vi "main.vi"() -> ()   [LabVIEW 2010]
uses:
  scan_specification_tagResonant.ctl
  common_typedefs/DAC_voltage_tagResonantr.ctl
  FPGA tracking/polar tracking settings.ctl
  FPGA tracking/spot location constraints.ctl
  FPGA tracking/spot location constraint.ctl
  FPGA tracking/kalman N spot state.ctl
  counter_cluster_tagResonant.ctl
  integration_cluster.ctl
  common_typedefs/channels_cluster.ctl
  FPGA tracking/kalman pv state.ctl
  FPGA tracking/control flags.ctl
  <vilib>/Platform/TimedLoop/XDataNode/XDataNode.xnode
  <vilib>/Platform/TimedLoop/XDataNode/timing_clust.ctl
  <vilib>/Platform/TimedLoop/XDataNode/nitl_modes.ctl
  <vilib>/Platform/TimedLoop/XDataNode/wakeup.ctl
  <vilib>/rvi/FXPMathLib/FxpMul/XNode/nifxpmath_Multiplier.xnode
  <vilib>/rvi/FXPMathLib/FxpMul/subVIs/nifxpmath_Mul_SimConfig.ctl
  <vilib>/fxp/LVFixedPointQuantizationPolicyTypeDef.ctl
  <vilib>/fxp/LVFixedPointOverflowPolicyTypeDef.ctl
  <vilib>/eio/EIONode/EIONode.xnode
  <vilib>/rvi/eio/nirviEIOImplementation/nirviEIOImplementation.xnode
  <vilib>/rvi/eio/common/nirviEmuClasses.ctl
  <vilib>/rvi/DataTransferAndStorage/Container/XNode/niFpgaContainer.xnode
  FPGA scanInfo/scan message.ctl
  <vilib>/rvi/DataTransferAndStorage/Container/Common/niFpgaContainerMethod.ctl
  <vilib>/rvi/DataTransferAndStorage/Container/Common/niFpgaTransferTypeControl.ctl
  <vilib>/rvi/FXPMathLib/FxpMul/simVIs/DllFxpMulTemp_sub.vi
  <vilib>/rvi/eio/common/nirviEmuTemplateMethod_noerrors.vi
  <vilib>/rvi/FIFO/Fifo_Resource/nirvififoEmulationSetSize.vi
  <vilib>/rvi/DataTransferAndStorage/Container/Common/niFpgaContainerGetUniqueNameForEmu.vi
  <vilib>/rvi/interface/RandomDataEmulation/nirviRandomDataFPGAFIFO.vi
  <vilib>/rvi/interface/RandomDataEmulation/niFpgaRandomDataHandleErrors.vi
  <vilib>/Platform/TimedLoop/XDataNode/XDNodeRunTimeDep.lvlib
panel:
  in  "total cycles per stim cycle":u16
  in  "lines per stim":u16
  in  "stim by cycle":bool
  in  "stim delay":i16=5
  in  "bleach mode":bool
  in  "pockels always on":bool
  in  "invert optog stim":bool
  in  "optog all spots":bool
  in  "optog target spot":u8
  in  "ff vel?":bool
  out "N spot tracker out":T1
  in  "spot location constraints":T2=[{"spot number"=0, "active"=FALSE, "x max"=0, "x min"=0, "y max"=0, "y min"=0}, {"spot number"=0, "active"=FALSE, "x max"=0, "x min"=0, "y max"=0, "y min"=0}, {"spot number"=0, "active"=FALSE, "x max"=0, "x min"=0, "y max"=0, "y min"=0}, {"spot number"=0, "active"=FALSE, "x max"=0, "x min"=0, "y max"=0, "y min"=0}]
  in  "reset flags":u8
  in  "mark valid location":bool
  out "Spot locations":T4(array[cluster])
  in  "inter-spot delay":u8
  in  "circles per spot":u16
  in  "number of spots":u8
  in  "stim buffer counts":u16=20
  in  "TAG slice options":T5
  out "n photons during stim":u32
  out "stim time":u32
  in  "stimulus on (low f)":bool=TRUE
  out "y-offset":i16
  out "x-offset":i16
  in  "measure offset":bool
  in  "Vxy feedback":bool
  out "piezo z-offset":i16
  in  "piezoToTrackingScale":fxp<+/-,16,2>
  out "piezo out":i16
  in  "piezo z feedback":bool
  in  "trackingToPiezoScale":fxp<+/-,16,5> format="%.16g"
  out "z-location":i16
  in  "Vz feedback?":bool
  in  "half valid z-range (ncycles * 64)":i16=500
  in  "x-y phase shift (*2^16/2*pi)":u16=16384
  in  "vmax":fxp<+,16,0>=0.0016021728515625 format="%.32g"
  in  "tracking settings":T6
  out "AI values":u32
  in  "min photons for update":u32=200
  out "pixels sent":u32
  out "lines sent":u32
  in  "tracking?":bool
  in  "feedback channel":enum16{"channel 0", "channel 1", "both"}(ring)=enum."both"
  out "ticks for AI read":u32
  in  "AI look-ahead":i16
  out "ticks to transmit":i32
  in  "useReadPosition":bool
  out "DAC voltages":T7 {"pockels" max=4095 step=1; "y" max=4095 step=1; "x" max=4095 step=1}
  in  "scan specification":T8={"z resolution (pixels)"=1000, "iterations per pixel"=28, "iterations per z-scan (=zres*iterperpixel)"=50, "x resolution (pixels)"=100, "y resolution (pixels)"=80, "number of z-lines per volume"=30, "number of repetitions (volumes)"=5, "Pockels cell voltage (bits)"=-1, "Vx center (bits)"=0, "Vy center (bits)"=0, "Vx amplitude (bits)"=40, "Vy amplitude (bits)"=0, "lines to delay between scan start and output"=1, "LSB has acquire control"=FALSE, "Pockels cell bleach voltage"=0}
  out "FIFO overflow":bool
  in  "scan":bool
  in  "stop":bool
  in  "stop acquisition at\nFIFO overflow?":bool
  out "scanning?":bool
  # "Mirna: \niterations per pixel = (x scan segment fraction*fFPGA)/(x resolution*f resonance)\nfFPGA/f resonance = 5000 --assumes 8kHz resonance frequency\niterations per pixel=25"
  # "used to be 1000 (Mirna)"
  # "to control how line locations are found"
  # "y settings:\ny resolution*y step size = 6553\nthis gives scan from -1 to 1V\ny resolution = 200\ny step size = 33\n\nz settings:\nto scan entire y profile \nnumber of z's has to be equal\ny resolution"
  # "1. use ftn generators to test galvo inputs\n2. right now AI+ and AI- == differential configuration\nThere is also an option AI+ and GND = referenced single ended"
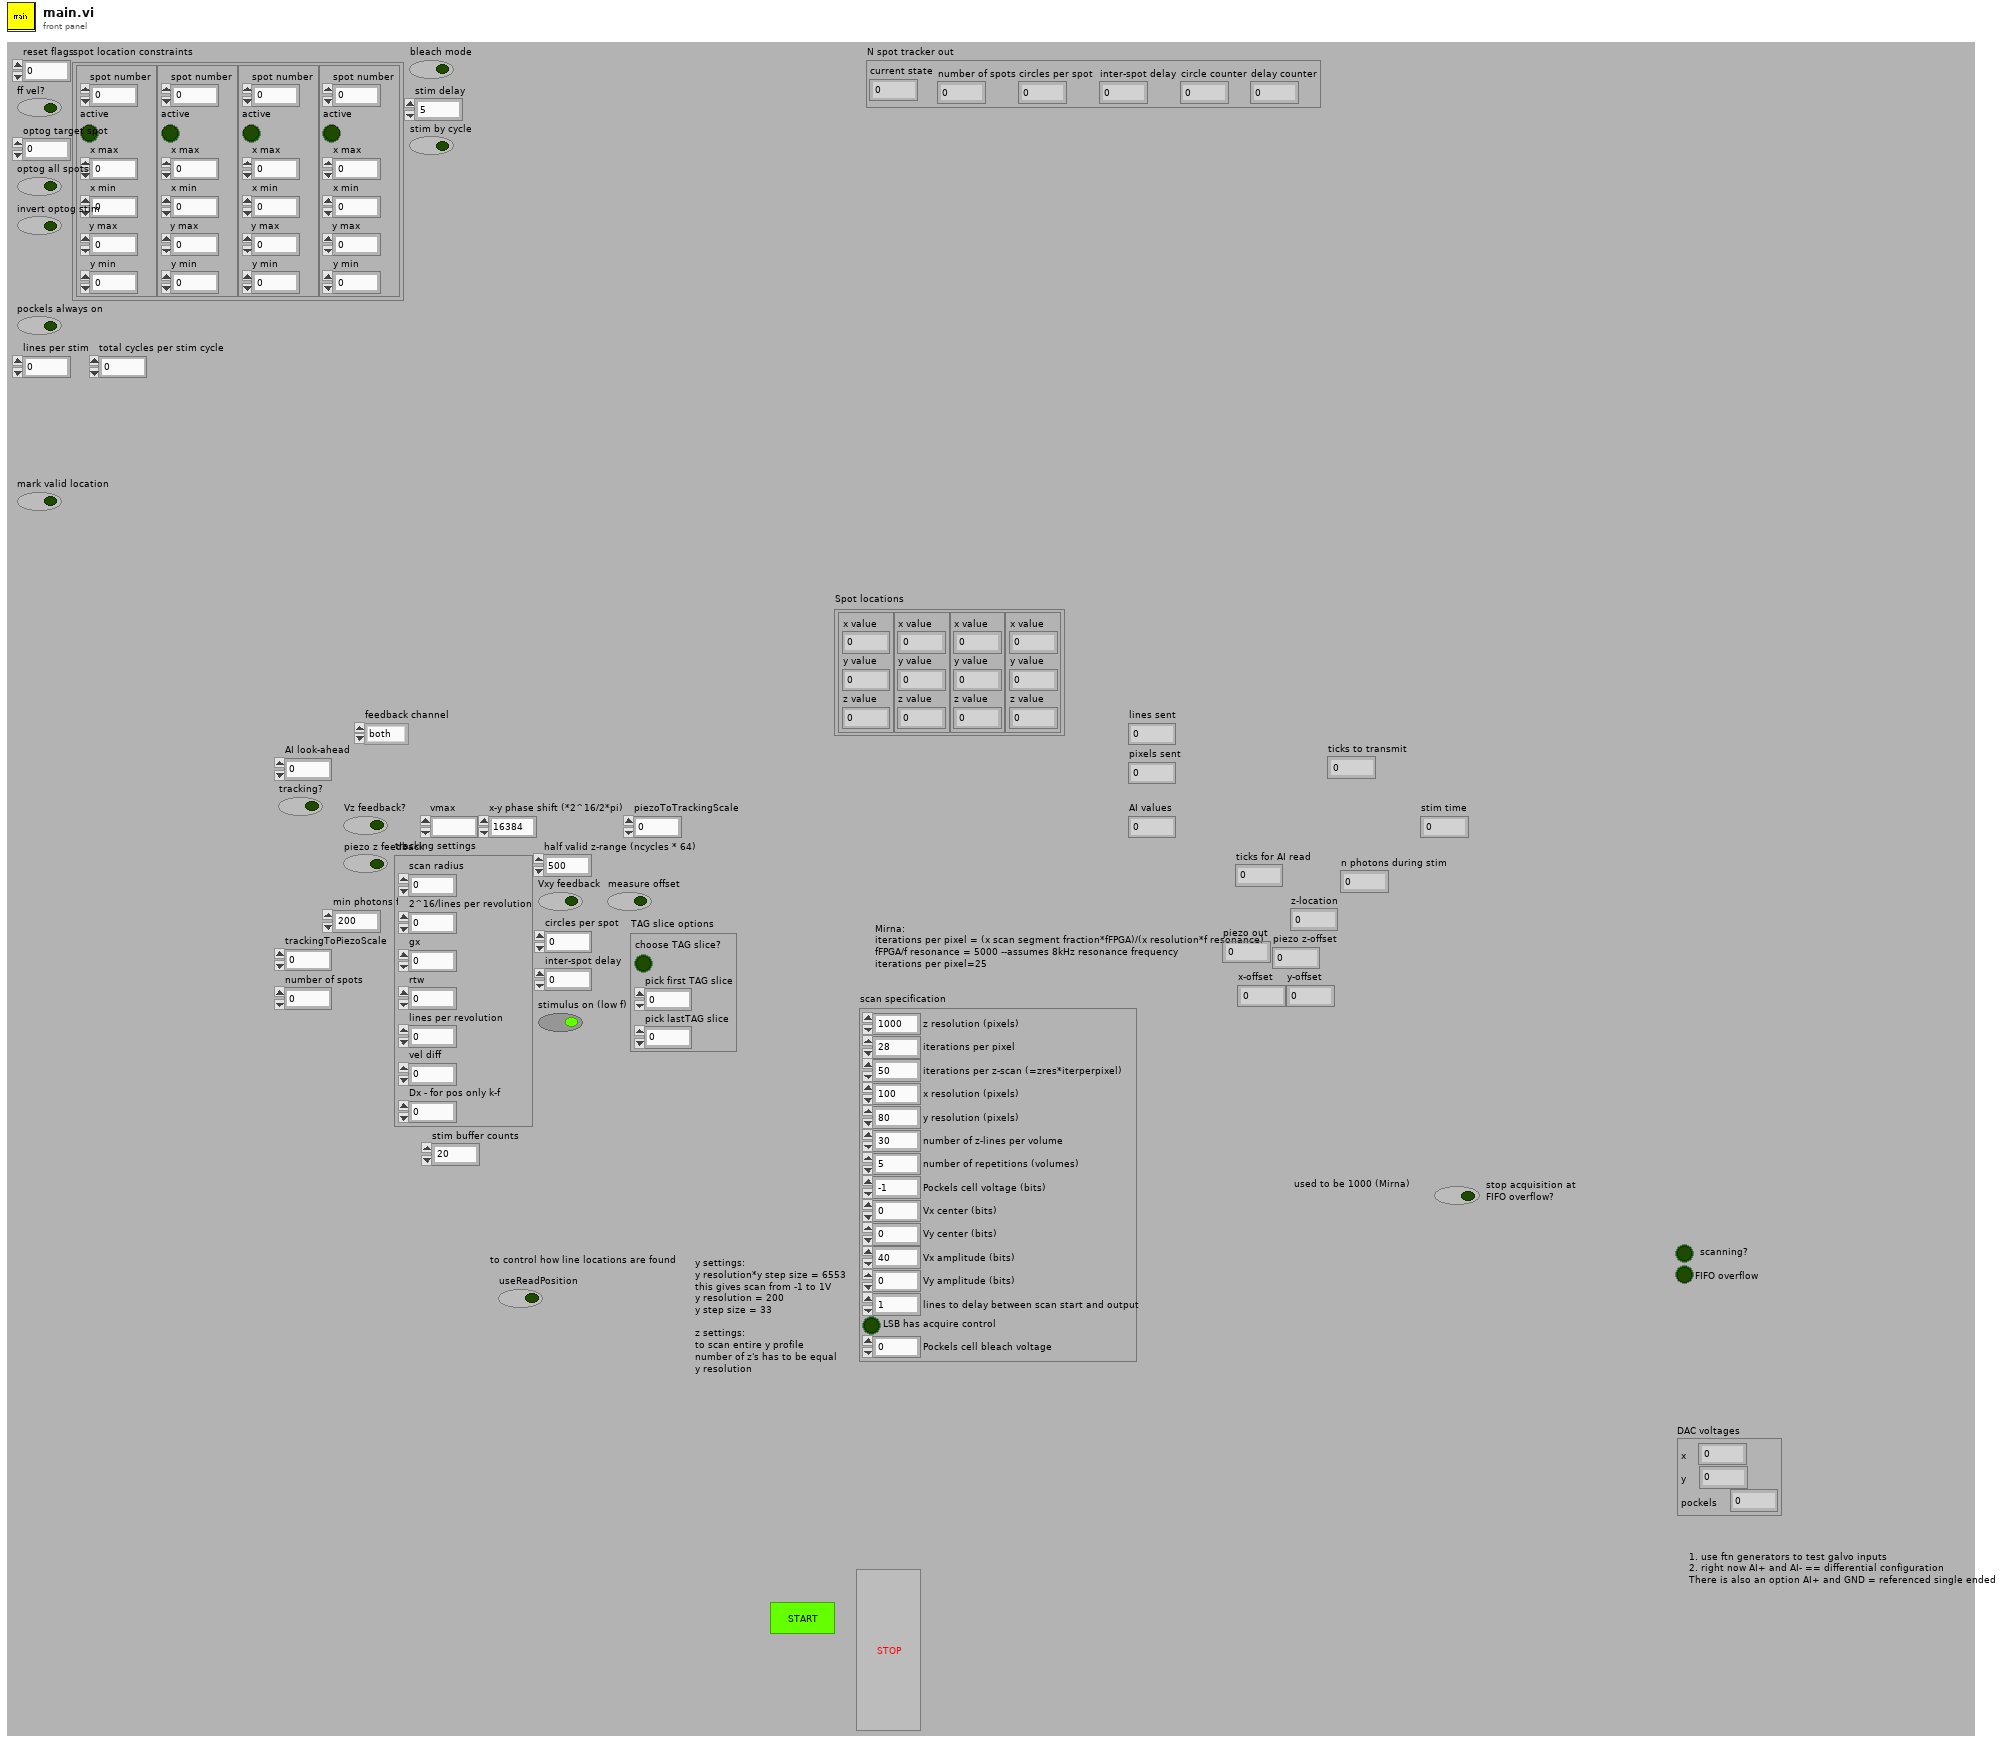
[diagram p1: front panel]
types:
  T1 = typedef "kalman N spot state.ctl" = cluster{"current state":u8, "number of spots":u8, "circles per spot":u16, "inter-spot delay":u8, "circle counter":u16, "delay counter":u8}
  T2 = typedef "spot location constraints.ctl" = T3[]
  T3 = typedef "spot location constraint.ctl" = cluster{"spot number":i8, "active":bool, "x max":i16, "x min":i16, "y max":i16, "y min":i16}
  T4 = cluster{"x value":i16, "y value":i16, "z value":i16}[]
  T5 = cluster{"choose TAG slice?":bool, "pick first TAG slice":u32, "pick lastTAG slice":u32}
  T6 = typedef "polar tracking settings.ctl" = cluster{"scan radius":u16, "2^16/lines per revolution":u16, "gx":fxp<+,16,8>, "rtw":fxp<+,16,26>, "lines per revolution":u8, "vel diff":fxp<+,24,-22>, "Dx - for pos only k-f":fxp<+,32,19>}
  T7 = typedef "DAC_voltage_tagResonantr.ctl" = cluster{"x":i16, "y":i16, "pockels":i16}
  T8 = typedef "scan_specification_tagResonant.ctl" = cluster{"z resolution (pixels)":u16, "iterations per pixel":u16, "iterations per z-scan (=zres*iterperpixel)":u16, "x resolution (pixels)":u16, "y resolution (pixels)":u16, "number of z-lines per volume":u16, "number of repetitions (volumes)":i32, "Pockels cell voltage (bits)":i16, "Vx center (bits)":i16, "Vy center (bits)":i16, "Vx amplitude (bits)":i16, "Vy amplitude (bits)":i16, "lines to delay between scan start and output":u16, "LSB has acquire control":bool, "Pockels cell bleach voltage":i16}
  T9 = typedef "control flags.ctl" = cluster{"scanning":bool, "tracking?":bool, "acquire?":bool, "counting photons?":bool, "fly-back acquisition phase?":bool, "stim light window":bool, "use photons for tracking":bool}
  T10 = typedef "kalman pv state.ctl" = cluster{"estimates":cluster{"x":fxp<+/-,18,16>, "v":fxp<+/-,18,16>, "pxx":u16, "pxv":u16, "pvv":u16}, "model params":cluster{"qxx":u16, "qxv":u16, "qvv":u16, "r":u16}}
  T11 = typedef "channels_cluster.ctl" = cluster{"channel 0":u32, "channel 1":u32, "channel 2":u32, "channel 3":u32}
  T12 = typedef "integration_cluster.ctl" = cluster{"channel 0":u32, "channel 1":u32, "fly-back heap address":u32}
  T13 = typedef "counter_cluster_tagResonant.ctl" = cluster{"iteration counter (pixel)":u16, "pixel counter":u16, "line counter":i16, "volumes counter":u16}
  T14 = typedef "XDNodeRunTimeDep.lvlib/timing_clust.ctl" = cluster{"Expected End [f-1]":u64, "Actual End [f-1]":u64, "Finished Late? [f-1]":bool, "Expected End [i-1]":u64, "Actual End [i-1]":u64, "Finished Late? [i-1]":bool, "Expected Start [i]":u64, "Actual Start [i]":u64, "Expected Start [f]":u64, "Actual Start [f]":u64, "Source Name":string, "Structure Name":string, "Period":i64, "Deadline":i64, "Offset":i64, "Start":i64, "Priority":i32, "Timeout":i32, "Mode":T15, "Wakeup Reason":T16, "Error":errorcluster, "Source Type":string, "Secondary Source Type":string, "Global End Time":u64, "Global Start Time":u64, "Frame Duration":u64, "Iteration Duration":u64, "Assigned CPU":i32, "I/O Scan Engine Mode":u32}
  T15 = typedef "XDNodeRunTimeDep.lvlib/nitl_modes.ctl" = enum32{"No Change", "Process missed periods, maintain original phase", "Discard missed periods, maintain original phase", "Process missed periods, ignore original phase", "Discard missed periods, ignore original phase"}
  T16 = typedef "XDNodeRunTimeDep.lvlib/wakeup.ctl" = enum32{"Normal", "Aborted", "Asynchronous wakeup", "Timing source error", "Timed loop error", "Timeout"}
  T17 = cluster{"pos estimate":fxp<+/-,32,16>, "v estimate":fxp<+/-,16,0>, "weighted position error sum":fxp<+/-,32,32>, "photon count":u32, "transmit tick count":u32, "axis number":u8, "px (levels^2)":fxp<+,32,19>, "pxv (levels^2/ticks)":fxp<+,32,2>, "pv (levels^2/ticks^2)":fxp<+,32,-14>, "vel diff (levels^2/ticks^3)":fxp<+,24,-22>, "gx":fxp<+,16,8>, "rtwiddle":fxp<+,16,26>, "photon count ch0":u32, "photon count ch1":u32, "Dx - for pos only k-f":fxp<+,32,19>}
  T18 = typedef "integrating single axis kalman state.ctl" = cluster{"pos estimate":fxp<+/-,32,16>, "v estimate":fxp<+/-,16,0>, "weighted position error sum":fxp<+/-,32,32>, "photon count":u32, "transmit tick count":u32, "axis number":u8, "px (levels^2)":fxp<+,32,19>, "pxv (levels^2/ticks)":fxp<+,32,2>, "pv (levels^2/ticks^2)":fxp<+,32,-14>, "vel diff (levels^2/ticks^3)":fxp<+,24,-22>, "gx":fxp<+,16,8>, "rtwiddle":fxp<+,16,26>, "photon count ch0":u32, "photon count ch1":u32, "Dx -levels^2/ticks":fxp<+,32,19>}
  T19 = typedef "nirviEmuClasses.ctl" = enum16{"IO Read", "IO Write", "Method", "Property Read", "Property Write"}
  T20 = cluster{"stim by cycle":bool, "stim enable":bool, "lines per stim":u16, "total cycles per stim cycle":u16}
  T21 = cluster{"Kalman State":T18, "Kalman Update":bool}
  T22 = typedef "kalman 3-axis state.ctl" = cluster{"x state":T18, "y state":T18, "z state":T18, "spot number":u8}
  T23 = cluster{"x value":i16, "y value":i16, "z value":i16}
  T24 = typedef "scan_command.ctl" = cluster{"code":i32, "xdata":i32, "ydata":i32, "zdata":i32, "volume number":i32}
  T25 = typedef "scan message.ctl" = enum8{"NONE", "VOLUME START", "LINE START", "LINE START TRACKING", "XKALMAN", "YKALMAN", "ZKALMAN"}
  T26 = typedef "niFpgaContainerMethod.ctl" = enum16{"<none>", "write", "read", "clear", "getNumberOfElementsToWrite", "getNumberOfElementsToRead", "enable", "disable", "flushAndDisable", "getStreamState", "readA", "readB", "dramWrite", "dramWriteWithByteEnables", "dramRequestData", "dramRetrieveData"}
  T27 = typedef "niFpgaTransferTypeControl.ctl" = enum16{"Target-Scoped", "Host to Target - DMA", "Target to Host - DMA", "Peer to Peer Reader", "Peer to Peer Writer", "Bidirectional"}
  T28 = cluster{"code":i32, "xdata":i32, "ydata":i32, "zdata":i32, "volume number":i32}
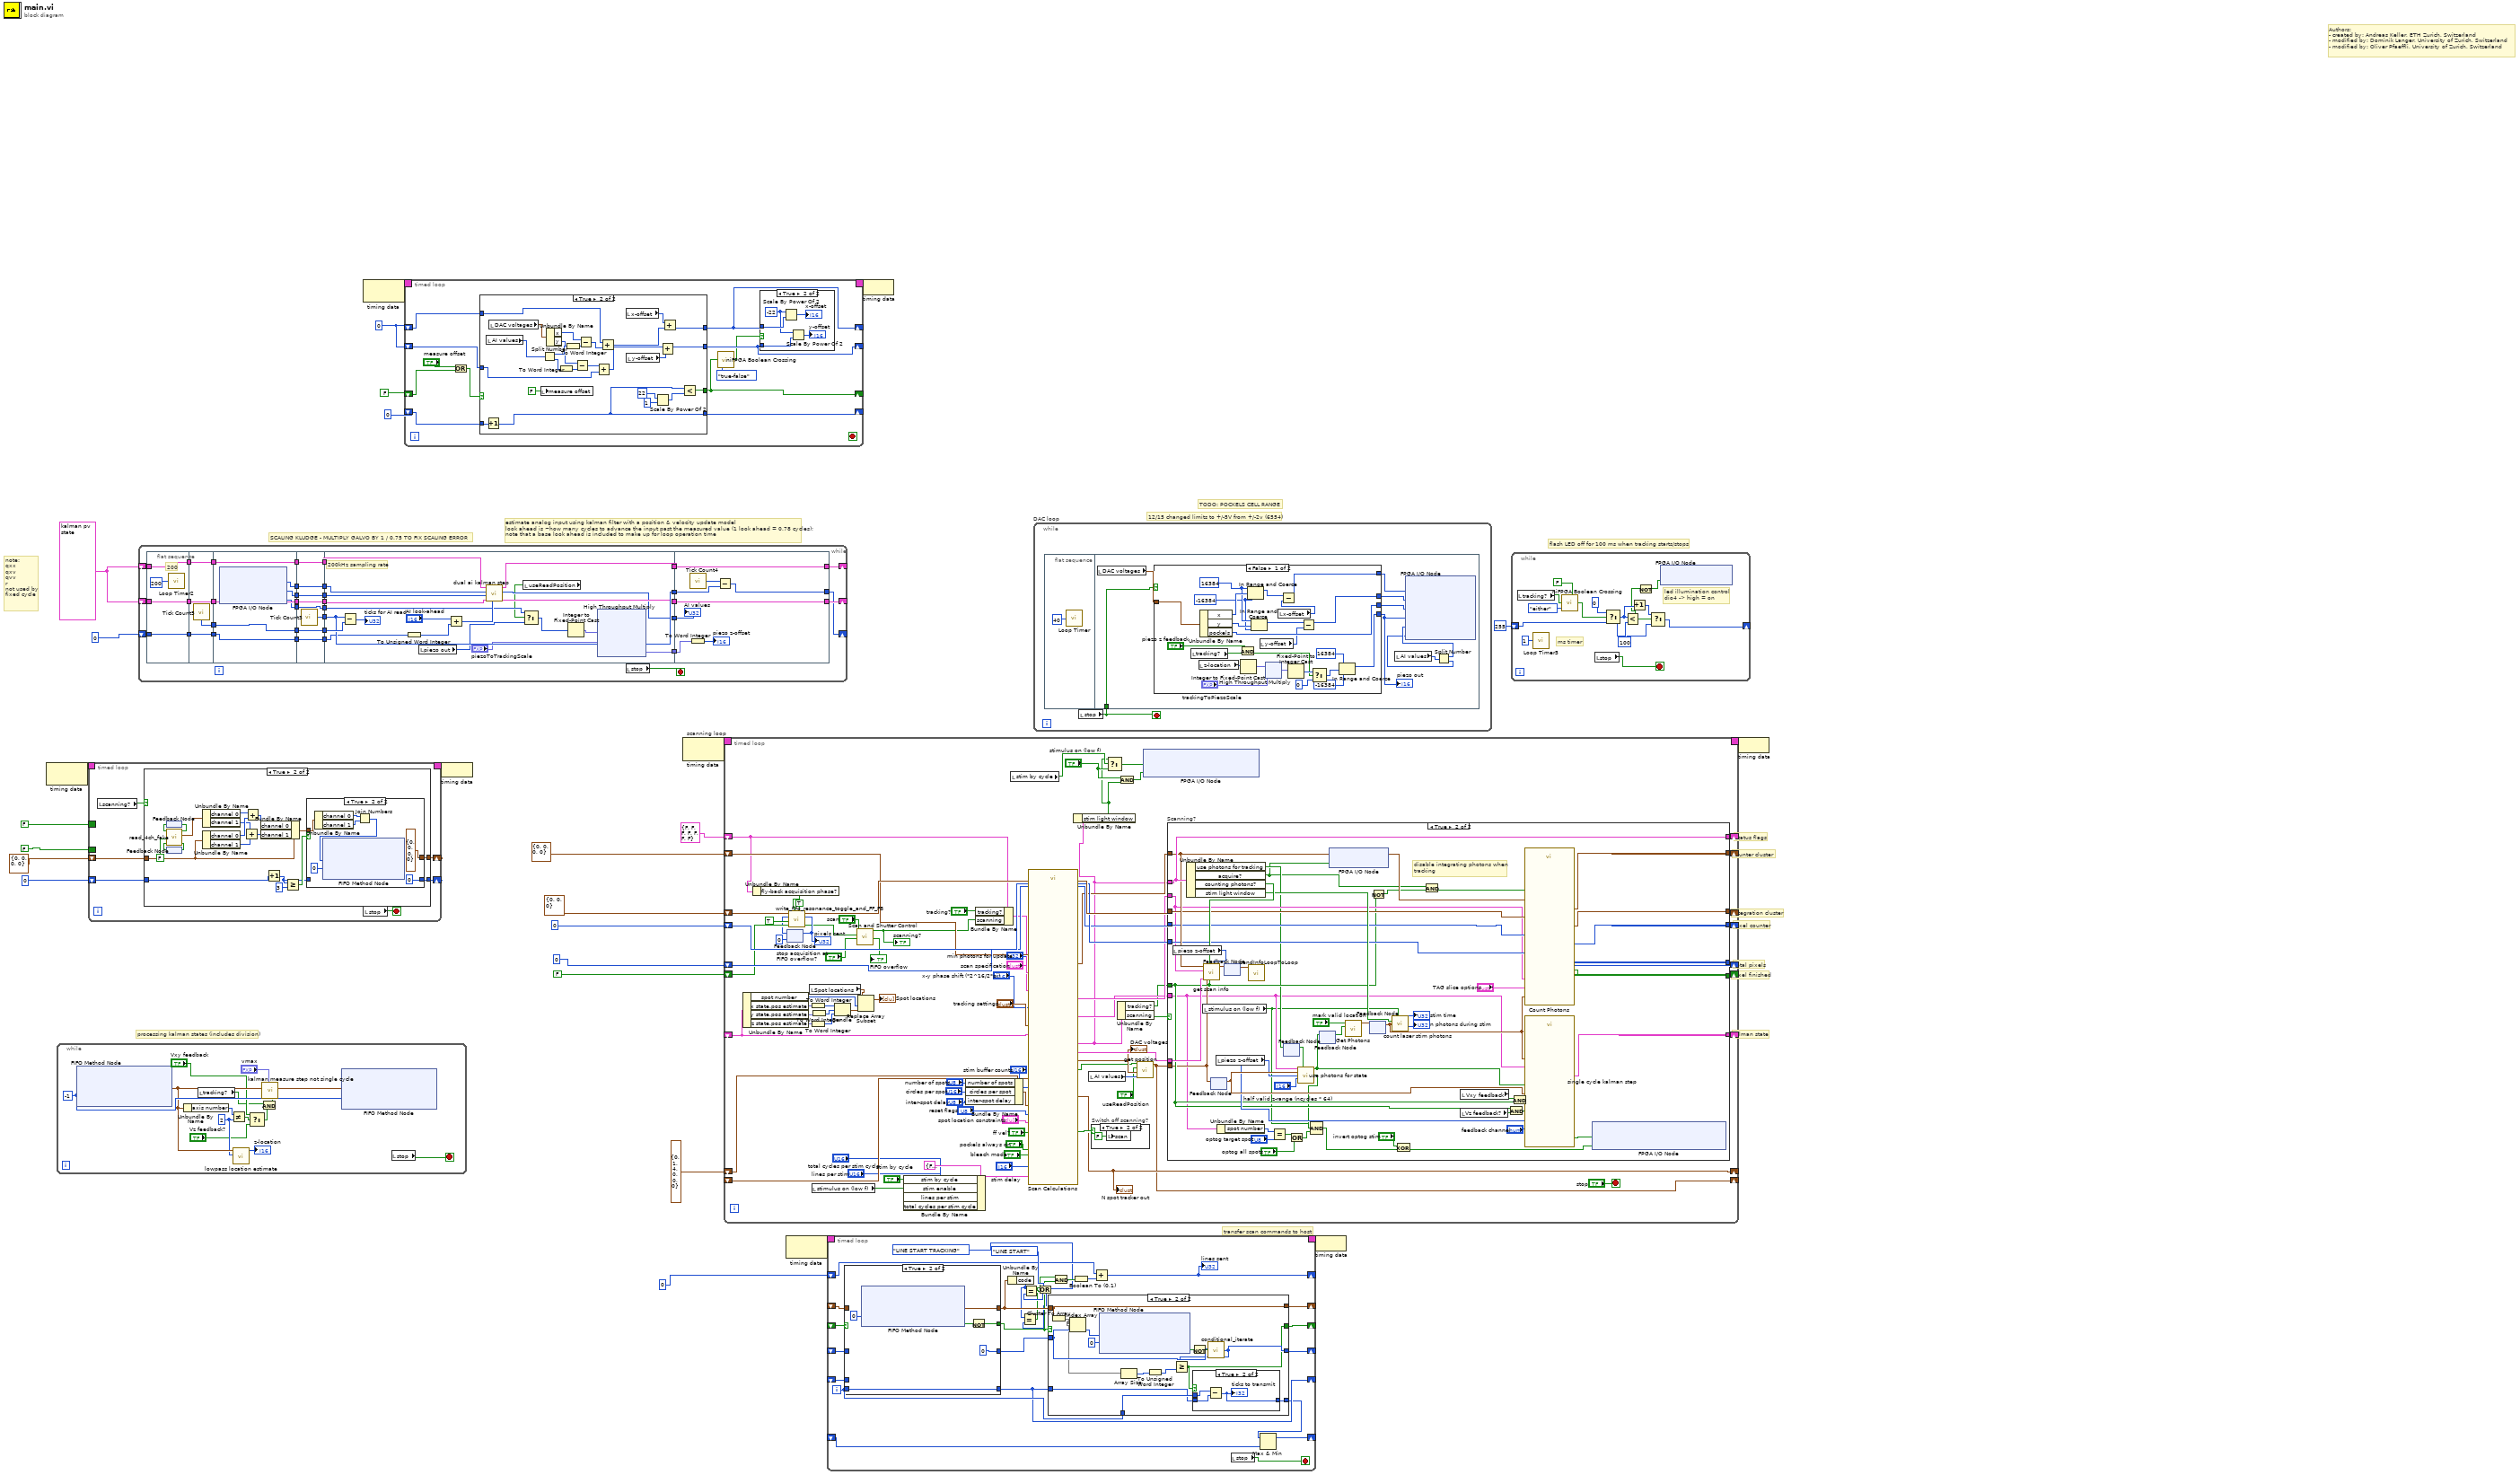
[diagram p0: block diagram]
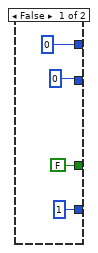
[diagram p3: hidden frame]
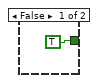
[diagram p4: hidden frame]
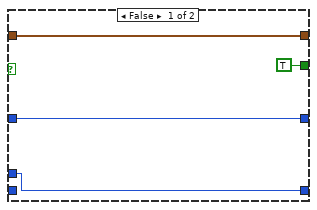
[diagram p6: hidden frame]
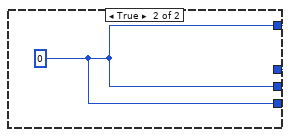
[diagram p9: hidden frame]
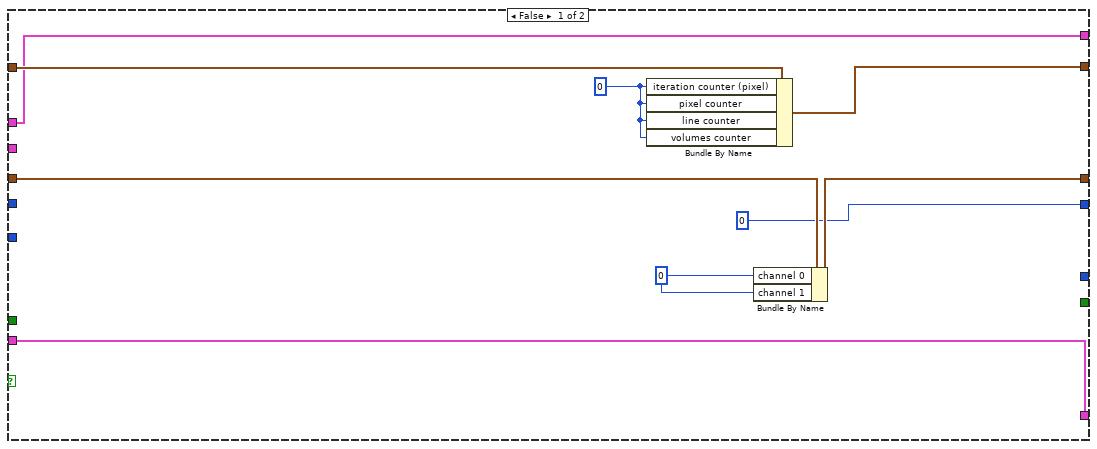
[diagram p11: hidden frame]
diagram:
  w5 = 0
  w11 = T10 {"estimates"={"x"=0.0, "v"=0.0, "pxx"=0, "pxv"=0, "pvv"=0}, "model params"={"qxx"=1, "qxv"=2, "qvv"=4, "r"=100}} ("kalman pv state out")
  # "status flags"
  # "flash LED off for 100 ms when tracking starts/stops"
  # "12/15 changed limits to +/-5V from +/-2v (6554)"
  # "note:\nqxx\nqxv\nqvv\nr\nnot used by\nfixed cycle"
  # "processing kalman states (includes division)"
  # "TODO: POCKELS CELL RANGE"
  # "kalman state"
  # "pixel finished"
  # "total pixels"
  # "pixel counter"
  # "integration cluster"
  # "counter cluster"
  # "estimate analog input using kalman filter with a position & velocity update model\nlook ahead is ~how many cycles to advance the input past the measured value (1 look ahead = 0.78 cycles);\nnote that a base look ahead is included to make up for loop operation time"
  # "SCALING KLUDGE - MULTIPLY GALVO BY 1 / 0.75 TO FIX SCALING ERROR"
  # "transfer scan commands to host"
  # "Authors: \n- created by: Andreas Keller, ETH Zurich, Switzerland\n- modified by: Dominik Langer, University of Zurich, Switzerland\n- modified by: Oliver Pfaeffli, University of Zurich, Switzerland"
  n1 = node-c288() -> (w20:T14)  [unwired: 1 in]
  n2 = while {
    stop <- w40 stop-if-true
    w33 = u8 2 ("y")
    w39 = -1 ("Timeout")
    n3 = xnode ("FIFO Method Node")("Timeout"=w39) -> ("Element"=w34:T17)  [unwired: 1 in, 2 out]
    n4 = Unbundle By Name(w34) -> ("axis number"=w36:u8)
    n5 = local read "tracking?"() -> (w27:bool)
    n6 = Not Equal?(x=w36, y=w33) -> (x != y?=w31:bool)
    n7 = call "lowpass location estimate.vi"("axis number"=w33, "kalman state"=w34) -> ("location"=→"z-location":i16)  [unwired: 9 in]
    n8 = Select(t="Vxy feedback", s=w31, f="Vz feedback?") -> (s? t:f=w35:bool)
    n9 = And(x=w27, y=w35) -> (x .and. y?=w28:bool)
    n10 = call "kalman measure step not single cycle.vi"("v-feedback?"=w28, "vmax"="vmax", "state in"=w34) -> ("state out"=w37:T18)  [unwired: 8 in]
    n11 = xnode ("FIFO Method Node")("Element"=w37, "Timeout"=w39) -> ()  [unwired: 1 in, 2 out]
    n12 = local read "stop"() -> (w40:bool)
  }
  n13 = timed-loop {
    timing: w20 -> [_]
    timing-out: [_] -> w19
    border: FALSE ("Input0") -> [_]
    border: FALSE ("Inputl1") -> [_]
    shift-right: [w146] -> _
    shift-left: T11 {"channel 0"=0, "channel 1"=0, "channel 2"=0, "channel 3"=0} ("read output") -> [w147]
    shift-right: [w144] -> _
    shift-left: u8 0 -> [w145]
    stop <- w143 stop-if-true
    n14 = local read "scanning?"() -> (w148:bool)
    n15 = case shown="True" w148 {
      tunnel: w147 -> [_ w159]
      tunnel: [_ w151] -> w146
      tunnel: w145 -> [_ w156]
      tunnel: [_ w153] -> w144
      frame False {
      }
      frame True {
        n16 = feedback #1() -> (w167:bool)
        n17 = feedback #2() -> (w166:bool)
        n18 = call "read_4ch_fake.vi"("previous value ch1"=w166, "fake image fast loop?"=FALSE, "previous value ch0"=w167) -> ("Inputl1"=w165:bool, "read output"=w149:T11, "Input0"=w168:bool)  [unwired: 6 in]
        n19 = feedback-in #1(w168) -> ()
        n20 = feedback-in #2(w165) -> ()
        n21 = Unbundle By Name(w149) -> ("channel 0"=w164:u32, "channel 1"=w162:u32)
        n22 = Unbundle By Name(w159) -> ("channel 0"=w163:u32, "channel 1"=w161:u32)
        n23 = Add(x=w162, y=w161) -> (x+y=w160:u32)
        n24 = Add(x=w164, y=w163) -> (x+y=w152:u32)
        n25 = Bundle By Name(cluster=w159, "channel 0"=w152, "channel 1"=w160) -> (w158:T11)
        n26 = Increment(x=w156) -> (x+1=w154:u8)
        n27 = Greater Or Equal?(x=w154, y=u8 3) -> (x >= y?=w155:bool)
        n28 = case shown="True" w155 {
          tunnel: [w170 T11 {"channel 0"=0, "channel 1"=0, "channel 2"=0, "channel 3"=0} ("read output")] -> w151
          tunnel: w158 -> [w170 w174]
          tunnel: w154 -> [w169 _]
          tunnel: [w169 u8 0] -> w153
          frame False {
          }
          frame True {
            n29 = Unbundle By Name(w174) -> ("channel 0"=w173:u32, "channel 1"=w172:u32)
            n30 = Join Numbers(hi=w173, lo=w172) -> ((hi.lo)=w171:u64)
            n31 = xnode ("FIFO Method Node")("Element"=w171, "Timeout"=0) -> ()  [unwired: 1 in, 2 out]
          }
        }
      }
    }
    n32 = local read "stop"() -> (w143:bool)
  }
  n33 = while {
    shift-right: [w263] -> _
    shift-left: w11 -> [w262]
    shift-right: [w261] -> _
    shift-left: w11 -> [w260]
    shift-right: [w239] -> _
    shift-left: u32 0 -> [w238]
    stop <- w264 stop-if-true
    n34 = flat-sequence {
      tunnel: [w267] -> w244
      tunnel: w262 -> [w267]
      tunnel: w260 -> [w266]
      tunnel: [w266] -> w242
      tunnel: w238 -> [w265]
      tunnel: [w265] -> w237
      tunnel: w244 -> [w272]
      tunnel: [w272] -> w243
      tunnel: w242 -> [w271]
      tunnel: [w271] -> w241
      tunnel: [w270] -> w240
      tunnel: w237 -> [w269]
      tunnel: [w269] -> w236
      tunnel: w243 -> [w279]
      tunnel: [w279] -> w257
      tunnel: w241 -> [w278]
      tunnel: [w278] -> w255
      tunnel: [w277] -> w253
      tunnel: [w276] -> w251
      tunnel: w240 -> [w275]
      tunnel: [w275] -> w248
      tunnel: w236 -> [w274]
      tunnel: [w274] -> w235
      tunnel: [w273] -> w232
      tunnel: w257 -> [w344]
      tunnel: [w344] -> w256
      tunnel: w255 -> [w343]
      tunnel: [w343] -> w254
      tunnel: w253 -> [w342]
      tunnel: [w342] -> w252
      tunnel: w251 -> [w341]
      tunnel: [w341] -> w250
      tunnel: [w340] -> w249
      tunnel: w248 -> [w339]
      tunnel: [w339] -> w247
      tunnel: w235 -> [w338]
      tunnel: [w338] -> w234
      tunnel: w232 -> [w337]
      tunnel: [w337] -> w231
      tunnel: w256 -> [w362]
      tunnel: w254 -> [w360]
      tunnel: [w361] -> w259
      tunnel: [w359] -> w258
      tunnel: w252 -> [w357]
      tunnel: w250 -> [w356]
      tunnel: w249 -> [w363]
      tunnel: w247 -> [w365]
      tunnel: [w358] -> w246
      tunnel: [w363] -> w245
      tunnel: w234 -> [w354]
      tunnel: [w349] -> w233
      tunnel: w231 -> [w347]
      tunnel: [w402] -> w261
      tunnel: [w403] -> w263
      tunnel: w259 -> [w403]
      tunnel: w258 -> [w402]
      tunnel: w246 -> [w401]
      tunnel: w245 -> [w399]
      tunnel: [w398] -> w239
      tunnel: w233 -> [w397]
      frame #0 {
        # "200"
        n35 = call "Loop Timer2"("Count(Ticks)"=u16 200) -> ()  [unwired: 1 out]
      }
      frame #1 {
        n36 = call "Tick Count5"() -> ("Tick Count(Ticks)"=w270:u32)
      }
      frame #2 {
        n37 = xnode "FPGA I/O Node"() -> ("Connector0/AI0"=w277:i16, "Connector0/AI2"=w276:i16, "Connector0/AI4"=w273:i16)  [unwired: 3 in, 3 out]
      }
      frame #3 {
        n38 = call "Tick Count3"() -> ("Tick Count(Ticks)"=w340:u32)
      }
      frame #4 {
        # "200kHz sampling rate"
        n39 = Subtract(x=w363, y=w365) -> (x-y=→"ticks for AI read":u32)
        n40 = To Unsigned Word Integer(number=w354) -> (unsigned 16bit integer=w353:u16)
        n41 = local read "piezo out"() -> (w348:i16)
        n42 = Add(x="AI look-ahead", y=w353) -> (x+y=w352:u16)
        n43 = call "dual ai kalman step.vi"("AI look-ahead"=w352, "y state in"=w360, "yval"=w356, "x val"=w357, "x state in"=w362) -> ("y state out"=w359:T10, "AI values"=w358:u32, "x state out"=w361:T10)  [unwired: 4 in]
        n44 = local read "useReadPosition"() -> (w346:bool)
        n45 = Select(t=w347, s=w346, f=w348) -> (s? t:f=w345:i16)
        n46 = Integer to Fixed-Point Cast(integer=w345) -> (fixed-point=w351:fxp<+/-,16,16>)  [unwired: 1 in]
        n47 = xnode "High Throughput Multiply"("x"=w351, "y"="piezoToTrackingScale") -> ("x*y"=w349:fxp<+/-,16,16>)
      }
      frame #5 {
        n48 = To Word Integer(number=w397) -> (16bit integer=→"piezo z-offset":i16)
        n49 = call "Tick Count4"() -> ("Tick Count(Ticks)"=w400:u32)
        n50 = Subtract(x=w400, y=w399) -> (x-y=w398:u32)
        "AI values" <- w401
      }
    }
    n51 = local read "stop"() -> (w264:bool)
  }
  n52 = node-c288() -> (w8:T14)  [unwired: 1 in]
  n53 = timed-loop {
    timing: w8 -> [_]
    timing-out: [_] -> w7
    shift-right: [w414] -> _
    shift-left: u32 0 -> [w413]
    shift-right: [w406] -> _
    shift-left: FALSE -> [w411]
    shift-right: [w408] -> _
    shift-left: w5 -> [w410]
    shift-right: [w407] -> _
    shift-left: w5 -> [w409]
    stop <- _ stop-if-true
    n54 = Or(x="measure offset", y=w411) -> (x .or. y?=w412:bool)
    n55 = case shown="True" w412 {
      tunnel: [u32 1 w428] -> w414
      tunnel: w413 -> [_ w449]
      tunnel: [FALSE w448] -> w406
      tunnel: [0 w431] -> w408
      tunnel: [0 w433] -> w407
      tunnel: w410 -> [_ w426]
      tunnel: w409 -> [_ w427]
      frame False {
      }
      frame True {
        n56 = Increment(x=w449) -> (x+1=w428:u32)
        n57 = local read "AI values"() -> (w447:u32)
        n58 = local read "DAC voltages"() -> (w446:T7)
        n59 = local write "measure offset"(FALSE ("measure offset")) -> ()
        n60 = Split Number(x=w447) -> (hi(x)=w444:u16, lo(x)=w441:u16)
        n61 = Unbundle By Name(w446) -> ("x"=w445:i16, "y"=w440:i16)
        n62 = To Word Integer(number=w441) -> (16bit integer=w442:i16)
        n63 = To Word Integer(number=w444) -> (16bit integer=w443:i16)
        n64 = Subtract(x=w440, y=w442) -> (x-y=w437:i16)
        n65 = Subtract(x=w445, y=w443) -> (x-y=w439:i16)
        n66 = Add(x=w437, y=w427) -> (x+y=w436:i32)
        n67 = Add(x=w426, y=w439) -> (x+y=w438:i32)
        n68 = local read "x-offset"() -> (w430:i16)
        n69 = local read "y-offset"() -> (w432:i16)
        n70 = Scale By Power Of 2(n=i8 22 ("y"), x=u32 1) -> (x*2^n=w429:u32)
        n71 = Add(x=w436, y=w432) -> (x+y=w433:i32)
        n72 = Add(x=w430, y=w438) -> (x+y=w431:i32)
        n73 = Less?(x=w428, y=w429) -> (x < y?=w448:bool)
      }
    }
    n74 = call <vilib>:"niFPGA Boolean Crossing.vi"("input"=w406, "direction"=enum8{"either", "false-true", "true-false"}."true-false") -> ("crossing"=w404:bool)  [unwired: 7 in]
    n75 = case shown="True" w404 {
      tunnel: w408 -> [_ w420]
      tunnel: w407 -> [_ w418]
      frame False {
      }
      frame True {
        w416 = -22 ("n")
        n76 = Scale By Power Of 2(n=w416, x=w420) -> (x*2^n=→"x-offset":i32)
        n77 = Scale By Power Of 2(n=w416, x=w418) -> (x*2^n=→"y-offset":i32)
      }
    }
  }
  n78 = node-c288(w19) -> ()
  n79 = node-c288() -> (w26:T14)  [unwired: 1 in]
  n80 = timed-loop "scanning loop" {
    timing: w26 -> [_]
    timing-out: [_] -> w25
    shift-right: [w520] -> _
    shift-left: T13 {"iteration counter (pixel)"=0, "pixel counter"=0, "line counter"=0, "volumes counter"=0} ("counter cluster") -> [w514]
    shift-right: [w529] -> _
    shift-left: T12 {"channel 0"=0, "channel 1"=0, "fly-back heap address"=0} ("integration cluster") -> [w526]
    shift-right: [w531] -> _
    shift-left: u64 0 -> [w527]
    shift-right: [w525] -> _
    shift-left: FALSE ("finished?") -> [w521]
    shift-right: [w524] -> _
    shift-left: u32 0 ("pixel counter out") -> [w523]
    shift-right: [w519] -> _
    shift-left: _ -> [w481]
    shift-right: [w498] -> _
    shift-left: T9 {"scanning"=FALSE, "tracking?"=FALSE, "acquire?"=FALSE, "counting photons?"=FALSE, "fly-back acquisition phase?"=FALSE, "stim light window"=FALSE, "use photons for tracking"=FALSE} ("control flags in") -> [w502]
    shift-right: [w490] -> _
    shift-left: T1 {"current state"=0, "number of spots"=1, "circles per spot"=4, "inter-spot delay"=0, "circle counter"=0, "delay counter"=0} ("N spot tracker out") -> [w485]
    shift-right: [w467] -> _
    shift-left: _ -> [w466]
    stop <- "stop" stop-if-true
    n81 = Unbundle By Name(w481) -> ("spot number"=w482:u8, "x state.pos estimate"=w480:fxp<+/-,32,16>, "y state.pos estimate"=w479:fxp<+/-,32,16>, "z state.pos estimate"=w478:fxp<+/-,32,16>)
    n82 = Unbundle By Name(w502) -> ("fly-back acquisition phase?"=w501:bool)
    n83 = feedback #3(u32 0 ("pixels sent out")) -> (w517:u32)
    n84 = call "write_fifo_resonance_toggle_and_FF_FB.vi"("enable fly-back reversion?"=TRUE, "fly-back?"=w501, "pixel finished?"=w521, "mark fly-back"=TRUE ("mark fly-back?"), "pixels sent in"=w517, "integration cluster in"=w526) -> ("FIFO overflow out"=w496:bool, "pixels sent out"=w518:u32, "integration cluster out"=w528:T12)  [unwired: 3 in]
    "pixels sent" <- w518
    n85 = feedback-in #3(w518) -> ()
    n86 = local read "Spot locations"() -> (w484:T4)
    n87 = To Word Integer(number=w478) -> (16bit integer=w475:i16)
    n88 = To Word Integer(number=w480) -> (16bit integer=w477:i16)
    n89 = To Word Integer(number=w479) -> (16bit integer=w476:i16)
    n90 = local read "stimulus on (low f)"() -> (w458:bool)
    n91 = Bundle(w477, w476, w475) -> (w474:cluster{i16, i16, i16})  [unwired: 1 in]
    n92 = call "Scan and Shutter Control.vi"("stop acquisition at\nFIFO overflow?"="stop acquisition at\nFIFO overflow?", "fifo overflow in"=w496, "scan"="scan") -> ("FIFO overflow"=→"FIFO overflow":bool, "scanning?"=w493:bool)  [unwired: 7 in]
    "scanning?" <- w493
    n93 = Replace Array Subset(array=w484, new element=w474, index=w482) -> (→"Spot locations":T4)
    n94 = Bundle By Name(cluster=T20 {"stim by cycle"=FALSE, "stim enable"=FALSE, "lines per stim"=42, "total cycles per stim cycle"=10} ("stim by cycle settings"), "stim by cycle"="stim by cycle", "stim enable"=w458, "lines per stim"="lines per stim", "total cycles per stim cycle"="total cycles per stim cycle") -> (w460:T20)
    n95 = Bundle By Name(cluster=w485, "number of spots"="number of spots", "circles per spot"="circles per spot", "inter-spot delay"="inter-spot delay") -> (w489:T1)
    n96 = Bundle By Name(cluster=w502, "tracking?"="tracking?", "scanning"=w493) -> (w509:T9)
    n97 = local read "stim by cycle"() -> (w453:bool)
    n98 = call "Scan Calculations.vi"("counter cluster in"=w514, "control flags in"=w509, "bleach mode"="bleach mode", "N spot tracker in"=w489, "scan specification in"="scan specification", "tracking settings"="tracking settings", "ff vel?"="ff vel?", "3-axis PV tracking state in"=w481, "x-y phase shift (*2^16/2*pi)"="x-y phase shift (*2^16/2*pi)", "min photons for update"="min photons for update", "reset flags"="reset flags", "spot location constraints"="spot location constraints", "pockels always on"="pockels always on", "current location"=w466, "stim duration"="stim buffer counts", "stim by cycle settings"=w460, "stim delay"="stim delay") -> ("end scan"=w500:bool, "trigger out"=w468:bool, "kalman to host"=w511:T21, "counter cluster out"=w512:T13, "control flags out"=w499:T9, "N spot tracker out"=w490:T1, "scan specification out"=w510:T8, "DAC voltages"=w471:T7, "3-axis PV tracking state out"=w505:T22)  [unwired: 2 in]
    "DAC voltages" <- w471
    "N spot tracker out" <- w490
    n99 = Unbundle By Name(w499) -> ("stim light window"=w452:bool)
    n100 = local read "AI values"() -> (w470:u32)
    n101 = case "Switch off scanning?" shown="True" w500 {
      frame False {
      }
      frame True {
        n102 = local write "scan"(FALSE ("scan")) -> ()
      }
    }
    n103 = Select(t=w452, s=w453, f="stimulus on (low f)") -> (s? t:f=w455:bool)
    n104 = Unbundle By Name(w499) -> ("tracking?"=w492:bool, "scanning"=w513:bool)
    n105 = And(x="stimulus on (low f)", y=w452) -> (x .and. y?=w515:bool)
    n106 = call "get position.vi"("AI values"=w470, "DAC voltages"=w471, "useReadPosition"="useReadPosition", "tag lens trigger"=w468) -> ("current location"=w467:T23)  [unwired: 6 in, 1 out]
    n107 = xnode "FPGA I/O Node"("Connector0/DIO13 (stim on)"=w455, "Connector0/DIO15 (stim window)"=w515) -> ()  [unwired: 2 in, 2 out]
    n108 = case "Scanning?" shown="True" w513 {
      tunnel: w512 -> [w560 w604]
      tunnel: w528 -> [w563 w602]
      tunnel: [w562 w601] -> w529
      tunnel: w510 -> [_ w596]
      tunnel: w527 -> [_ w598]
      tunnel: [_ w597] -> w531
      tunnel: [_ w594] -> w525
      tunnel: [u32 0 ("pixel counter out") w600] -> w524
      tunnel: w523 -> [_ w599]
      tunnel: [w559 w603] -> w520
      tunnel: [w558 w612] -> w519
      tunnel: w505 -> [w558 w576]
      tunnel: w511 -> [_ w614]
      tunnel: w492 -> [_ w579]
      tunnel: w499 -> [w556 w606]
      tunnel: [w556 w606] -> w498
      tunnel: w467 -> [_ w578]
      frame False {
        w557 = u16 0
        w564 = u32 0 ("channel 0")
        n109 = Bundle By Name(cluster=w560, "iteration counter (pixel)"=w557, "pixel counter"=w557, "line counter"=w557, "volumes counter"=w557) -> (w559:T13)
        n110 = Bundle By Name(cluster=w563, "channel 0"=w564, "channel 1"=w564) -> (w562:T12)
      }
      frame True {
        # "disable integrating photons when\ntracking"
        n111 = local read "piezo z-offset"() -> (w587:i16)
        n112 = Unbundle By Name(w606) -> ("use photons for tracking"=w577:bool, "acquire?"=w565:bool, "counting photons?"=w608:bool, "stim light window"=w607:bool)
        n113 = local read "stimulus on (low f)"() -> (w569:bool)
        n114 = call "get scan info.vi"("piezo z value"=w587, "tracking?"=w579, "counting photons?"=w608, "kalman to host"=w614, "current location"=w578, "scan specification"=w596, "counter cluster"=w604) -> ("scan info"=w616:T24)  [unwired: 4 in]
        n115 = feedback-in #4(w578) -> ()
        n116 = feedback #4() -> (w591:T23)  [unwired: 1 in]
        n117 = local read "piezo z-offset"() -> (w588:i16)
        n118 = Unbundle By Name(w576) -> ("spot number"=w575:u8)
        n119 = feedback-in #5(w616) -> ()
        n120 = feedback #5() -> (w615:T24)  [unwired: 1 in]
        n121 = call "sendInfoLoopToLoop.vi"("scan info"=w615) -> ()  [unwired: 8 in, 3 out]
        n122 = Equal?(x=w575, y="optog target spot") -> (x = y?=w573:bool)
        n123 = feedback-in #6(w577) -> ()
        n124 = feedback #6() -> (w589:bool)  [unwired: 1 in]
        n125 = Or(x=w573, y="optog all spots") -> (x .or. y?=w570:bool)
        n126 = call "use photons for state.vi"("state in"=w576, "apply measurement?"=w589, "location"=w591, "z-offset"=w588, "half valid z-range (ncycles * 64)"="half valid z-range (ncycles * 64)") -> ("use photons to update tracker?"=w583:bool, "on target"=w571:bool)  [unwired: 9 in]
        n127 = Compound Arithmetic op=AND(w569, w571, w570) -> (w568:bool)
        n128 = feedback-in #7(w583) -> ()
        n129 = feedback #7() -> (w582:bool)  [unwired: 1 in]
        n130 = xnode "FPGA I/O Node"("dio10 acquire"=w565) -> ()  [unwired: 1 in, 1 out]
        n131 = call "Get Photons.vi"("in range"=w582, "mark valid location"="mark valid location") -> ("read output"=w605:T11)  [unwired: 9 in]
        n132 = feedback #8() -> (w593:T11)  [unwired: 1 in]
        n133 = feedback-in #8(w605) -> ()
        n134 = Not(x=w579) -> (.not. x?=w585:bool)
        n135 = call "count laser stim photons.vi"("count window"=w569, "read output"=w593, "stim on?"=w607) -> ("n photons during stim"=→"n photons during stim":u32, "stim time"=→"stim time":u32)  [unwired: 7 in]
        n136 = Exclusive Or(1:w568, 2:"invert optog stim") -> (0:w567:bool)
        n137 = And(x=w565, y=w585) -> (x .and. y?=w586:bool)
        n138 = local read "Vz feedback?"() -> (w613:bool)
        n139 = local read "Vxy feedback"() -> (w611:bool)
        n140 = And(x=w579, y=w613) -> (x .and. y?=w580:bool)
        n141 = And(x=w611, y=w579) -> (x .and. y?=w581:bool)
        n142 = call "Count Photons.vi"("acquire?"=w586, "counter cluster in"=w604, "integration cluster in"=w602, "pixel counter in"=w599, "total pixels acquired in"=w598, "photon counts"=w593, "TAG slice options"="TAG slice options", "scan specifications"=w596) -> ("finished?"=w594:bool, "counter cluster out"=w603:T13, "integration cluster out"=w601:T12, "pixel counter out"=w600:u32, "total pixels acquired out"=w597:u64)  [unwired: 15 in]
        n143 = call "single cycle kalman step.vi"("state in"=w576, "apply measurement"=w583, "z-offset"=w588, "location"=w591, "pixel values cluster"=w593, "feedback channel"="feedback channel", "Vz feedback?"=w580, "Vxy feedback"=w581) -> ("state out"=w612:T22, "kalman counting"=w592:bool)  [unwired: 6 in]
        n144 = xnode "FPGA I/O Node"("Connector0/DIO12 counting kalman"=w592, "Connector0/DIO11 (optog stim window)"=w567) -> ()  [unwired: 2 in, 2 out]
      }
    }
  }
  n145 = node-c288() -> (w13:T14)  [unwired: 1 in]
  n146 = timed-loop {
    timing: w13 -> [_]
    timing-out: [_] -> w12
    shift-right: [w675] -> _
    shift-left: _ -> [w673]
    shift-right: [w677] -> _
    shift-left: _ -> [w672]
    shift-right: [w676] -> _
    shift-left: _ -> [w674]
    shift-right: [w670] -> _
    shift-left: _ -> [w669]
    shift-right: [w667] -> _
    shift-left: _ -> [w666]
    shift-right: [w658] -> _
    shift-left: u32 0 -> [w657]
    i -> [w671]
    stop <- w665 stop-if-true
    n147 = case shown="True" w674 {
      tunnel: [w728 w733] -> w664
      tunnel: [TRUE w730] -> w662
      tunnel: [w727 u16 0] -> w678
      tunnel: w673 -> [w728 _]
      tunnel: w672 -> [w727 _]
      tunnel: w671 -> [_ w729]
      tunnel: [w725 w729] -> w670
      tunnel: w669 -> [w725 _]
      frame False {
      }
      frame True {
        n148 = xnode ("FIFO Method Node")("Timeout"=0) -> ("Element"=w733:T28, "Timed Out?"=w732:bool)  [unwired: 1 in, 1 out]
        n149 = Not(x=w732) -> (.not. x?=w730:bool)
      }
    }
    n150 = Unbundle By Name(w664) -> ("code"=w656:i32)
    n151 = Equal?(x=w656, y=scan_message."LINE START TRACKING" ("Enum")) -> (x = y?=w653:bool)
    n152 = Equal?(x=w656, y=scan_message."LINE START" ("Enum")) -> (x = y?=w661:bool)
    n153 = Or(x=w653, y=w661) -> (x .or. y?=w654:bool)
    n154 = case shown="True" w662 {
      tunnel: w664 -> [_ w684]
      tunnel: w678 -> [_ w689]
      tunnel: [TRUE w683] -> w676
      tunnel: [_ w686] -> w677
      tunnel: [_ w684] -> w675
      tunnel: w670 -> [_ w681]
      tunnel: w671 -> [_ w682]
      tunnel: [_ w680] -> w668
      frame False {
      }
      frame True {
        n155 = Cluster To Array(cluster=w684) -> (array=w688:i32[])
        n156 = Index Array(array=w688, index=w689) -> (element=w693:i32)
        n157 = xnode ("FIFO Method Node")("Element"=w693, "Timeout"=0) -> ("Timed Out?"=w691:bool)  [unwired: 1 in, 1 out]
        n158 = Array Size(array=w688) -> (size(s)=w687:i32)
        n159 = To Unsigned Word Integer(number=w687) -> (unsigned 16bit integer=w685:u16)
        n160 = Not(x=w691) -> (.not. x?=w690:bool)
        n161 = call "conditional_iterate.vi"("iterate?"=w690, "number in"=w689) -> ("number out"=w686:u16)  [unwired: 4 in]
        n162 = Greater Or Equal?(x=w686, y=w685) -> (x >= y?=w683:bool)
        n163 = case shown="True" w683 {
          tunnel: w682 -> [_ w696]
          tunnel: w681 -> [_ w695]
          tunnel: [_ w694] -> w680
          frame False {
          }
          frame True {
            n164 = Subtract(x=w696, y=w695) -> (x-y=w694:i32)
            "ticks to transmit" <- w694
          }
        }
      }
    }
    n165 = And(x=w654, y=w662) -> (x .and. y?=w660:bool)
    n166 = Boolean To (0,1)(Boolean=w660) -> (0, 1=w659:i16)
    n167 = Add(x=w657, y=w659) -> (x+y=w658:u32)
    "lines sent" <- w658
    n168 = local read "stop"() -> (w665:bool)
    n169 = Max & Min(x=w668, y=w666) -> (max(x,y)=w667:i32)  [unwired: 1 out]
  }
  n170 = node-c288(w7) -> ()
  n171 = while "DAC loop" {
    stop <- w788 stop-if-true
    n172 = flat-sequence {
      tunnel: w788 -> [w797]
      frame #0 {
        n173 = call "Loop Timer"("Count(Ticks)"=u32 40) -> ()  [unwired: 1 out]
      }
      frame #1 {
        n174 = local read "DAC voltages"() -> (w798:T7)
        n175 = case shown="False" w797 {
          tunnel: w798 -> [w889 _]
          tunnel: [w868 w920] -> w796
          tunnel: [w866 w920] -> w795
          tunnel: [w871 w920] -> w794
          tunnel: [w870 w920] -> w793
          frame False {
            w885 = i16 -16384 ("lower limit")
            w886 = i16 16384 ("upper limit")
            n176 = local read "tracking?"() -> (w879:bool)
            n177 = local read "z-location"() -> (w884:i16)
            n178 = Unbundle By Name(w889) -> ("x"=w888:i16, "y"=w887:i16, "pockels"=w871:i16)
            n179 = And(x="piezo z feedback", y=w879) -> (x .and. y?=w877:bool)
            n180 = Integer to Fixed-Point Cast(integer=w884) -> (fixed-point=w883:fxp<+/-,16,16>)  [unwired: 1 in]
            n181 = In Range and Coerce(upper limit=w886, x=w888, lower limit=w885) -> (coerced(x)=w873:i16)  [unwired: 1 out]
            n182 = In Range and Coerce(upper limit=w886, x=w887, lower limit=w885) -> (coerced(x)=w872:i16)  [unwired: 1 out]
            n183 = local read "y-offset"() -> (w865:i16)
            n184 = xnode "High Throughput Multiply"("x"=w883, "y"="trackingToPiezoScale") -> ("x*y"=w881:fxp<+/-,16,16>)
            n185 = local read "x-offset"() -> (w867:i16)
            n186 = Subtract(x=w873, y=w867) -> (x-y=w868:i16)
            n187 = Fixed-Point to Integer Cast(1:w881) -> (0:w880:i16)
            n188 = Subtract(x=w872, y=w865) -> (x-y=w866:i16)
            n189 = Select(t=w880, s=w877, f=i16 0) -> (s? t:f=w869:i16)
            n190 = In Range and Coerce(upper limit=i16 16384, x=w869, lower limit=i16 -16384) -> (coerced(x)=w870:i16)  [unwired: 1 out]
          }
          frame True {
            w920 = i16 0 ("Connector0/AO0")
          }
        }
        "piezo out" <- w793
        n191 = local read "AI values"() -> (w792:u32)
        n192 = Split Number(x=w792) -> (hi(x)=w791:u16, lo(x)=w790:u16)
        n193 = xnode "FPGA I/O Node"("Connector0/AO0"=w796, "Connector0/AO1"=w795, "Connector0/AO4"=w794, "Connector0/AO3"=w793, "Connector0/AO6"=w791, "Connector0/AO7"=w790) -> ()  [unwired: 6 in, 6 out]
      }
    }
    n194 = local read "stop"() -> (w788:bool)
  }
  n195 = node-c288(w12) -> ()
  n196 = while {
    shift-right: [w926] -> _
    shift-left: u8 255 -> [w924]
    stop <- w921 stop-if-true
    # "led illumination control\ndio4 -> high = on"
    # "ms timer"
    n197 = local read "tracking?"() -> (w934:bool)
    n198 = call "Loop Timer3"("Count(mSec)"=u32 1) -> ()  [unwired: 1 out]
    n199 = call <vilib>:"niFPGA Boolean Crossing.vi"("input"=w934, "direction"=enum8{"either", "false-true", "true-false"}."either", "initialize"=FALSE) -> ("crossing"=w931:bool)  [unwired: 6 in]
    n200 = local read "stop"() -> (w921:bool)
    n201 = Select(t=u8 0, s=w931, f=w924) -> (s? t:f=w925:u8)
    n202 = Less?(x=w925, y=u8 100 ("led flash off duration")) -> (x < y?=w922:bool)
    n203 = Increment(x=w925) -> (x+1=w927:u8)
    n204 = Not(x=w922) -> (.not. x?=w923:bool)
    n205 = Select(t=w927, s=w922, f=w925) -> (s? t:f=w926:u8)
    n206 = xnode "FPGA I/O Node"("Connector0/DIO4"=w923) -> ()  [unwired: 1 in, 1 out]
  }
  n207 = node-c288(w25) -> ()
